vi "Revision Query.vi"(8 "error in (no error)":errorcluster, 11 "VISA resource name":refnum<visa-resource-name>) -> (0 "error out":errorcluster, 1 "Instrument Firmware Revision":string, 2 "Instrument Driver Revision":string, 3 "VISA resource name out":refnum<visa-resource-name>)   [LabVIEW 2017, in "HH PLI Series.lvlib"]
doc: "Queries the current instrument firmware revision and instrument driver revision.\n\nRefer to the Readme file for detailed driver information including modification history."
uses:
  HH PLI Series.lvlib
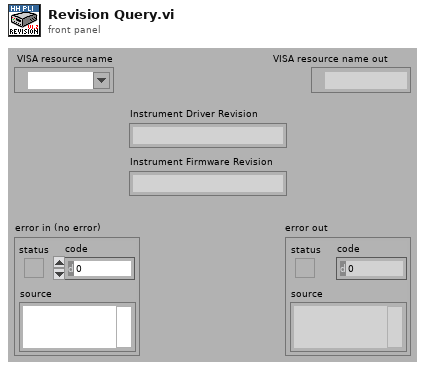
[diagram p1: front panel]
types:
  T1 = cluster{"Major":u16, "Minor":u16, "Fix":u16, "Build":u16}
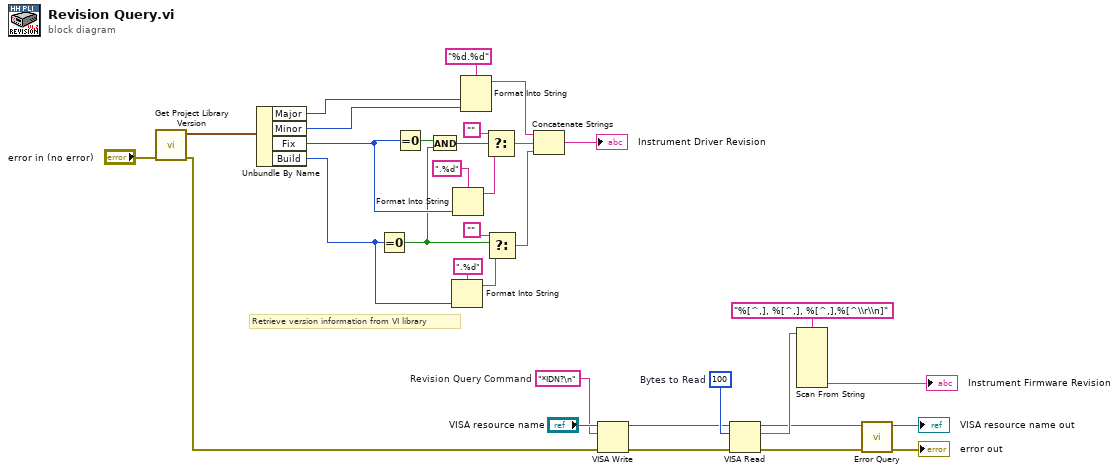
[diagram p0: block diagram]
diagram:
  w28 = "*IDN?\n"  # Revision Query Command
  w31 = u32 100  # Bytes to Read
  # "Retrieve version information from VI library"
  n1 = call <vilib>:"Get Project Library Version.vi"("error in (no error)"="error in (no error)") -> ("error out"=w3:errorcluster, "Project Library Version"=w4:T1)  [unwired: 9 in]
  n2 = Unbundle By Name(w4) -> ("Major"=w11:u16, "Minor"=w10:u16, "Fix"=w8:u16, "Build"=w9:u16)
  n3 = Equal To 0?(x=w9) -> (x = 0?=w6:bool)
  n4 = Equal To 0?(x=w8) -> (x = 0?=w7:bool)
  n5 = And(x=w7, y=w6) -> (x .and. y?=w5:bool)
  n6 = Format Into String(format string=".%d", w9) -> (resulting string=w15:string)  [unwired: 2 in, 1 out]
  n7 = Format Into String(format string=".%d", w8) -> (resulting string=w19:string)  [unwired: 2 in, 1 out]
  n8 = Format Into String(format string="%d.%d", w11, w10) -> (resulting string=w17:string)  [unwired: 2 in, 1 out]
  n9 = Select(t="", s=w5, f=w19) -> (s? t:f=w16:string)
  n10 = Select(t="", s=w6, f=w15) -> (s? t:f=w12:string)
  n11 = Concatenate Strings(w17, w16, w12) -> (→"Instrument Driver Revision":string)
  n12 = VISA Write(VISA resource name="VISA resource name", write buffer=w28, error in (no error)=w3) -> (VISA resource name out=w30:refnum<visa-resource-name>, error out=w29:errorcluster)  [unwired: 1 out]
  n13 = VISA Read(VISA resource name=w30, byte count=w31, error in (no error)=w29) -> (VISA resource name out=w24:refnum<visa-resource-name>, read buffer=w27:string, error out=w25:errorcluster)  [unwired: 1 out]
  n14 = Scan From String(format string="%[^,], %[^,], %[^,],%[^\\r\\n]", input string=w27) -> (output 4=→"Instrument Firmware Revision":string)  [unwired: 9 in, 3 out]
  n15 = call "Error Query.vi"("error in (no error)"=w25, "VISA resource name"=w24) -> ("error out"=→"error out":errorcluster, "VISA resource name out"=→"VISA resource name out":refnum<visa-resource-name>)  [unwired: 6 in, 2 out]
